vi "Project 5 Help 2.vi"() -> ()   [LabVIEW 2019]
panel:
  in  "stop":bool
  in  "stop (F)":bool
  out "size(s)":i32
  in  "Sim Mode":bool
  in  "Read File":bool
  out "Array":dbl[](array[numeric])
  out "Time":dynamicdata(graph)
  out "Data":dynamicdata(graph)
  out "Waveform Graph":waveform(dbl)(graph)
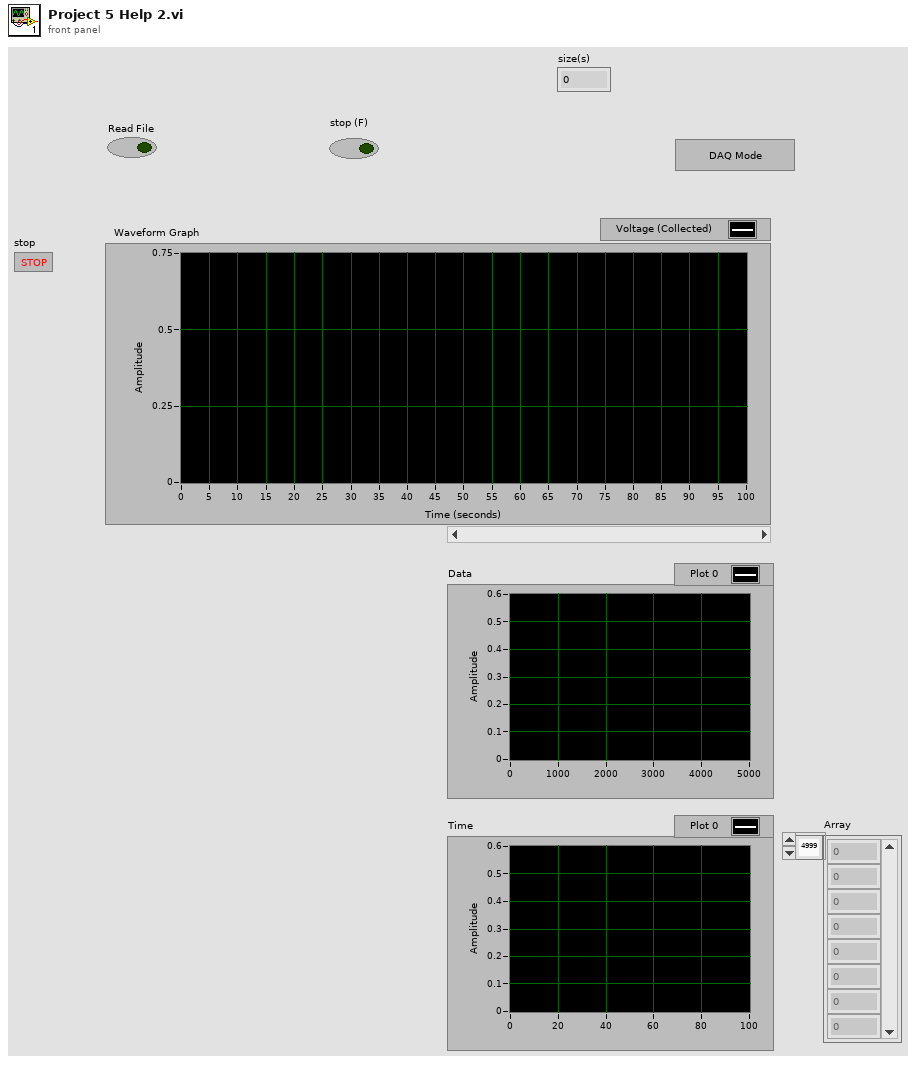
[diagram p1: front panel]
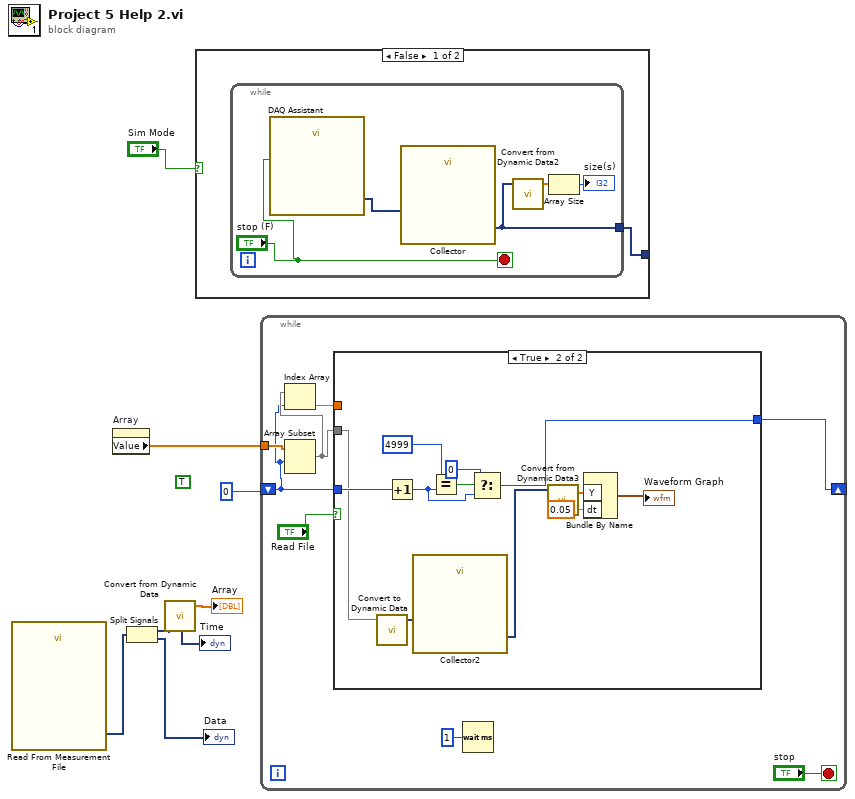
[diagram p0: block diagram]
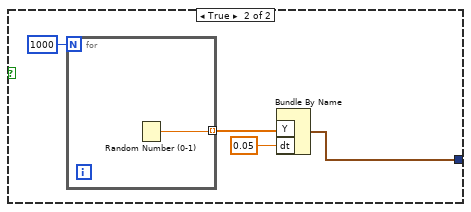
[diagram p3: hidden frame]
diagram:
  (unwired) TRUE ("EOF?")
  n1 = call "Read From Measurement File"() -> ("Signals"=w3:dynamicdata)  [unwired: 6 in, 5 out]
  n2 = property on="Array" class="Arr (strict)"() -> ("Value"=w2:dbl[])  [unwired: 2 in, 2 out]
  n3 = Split Signals(w3) -> (w5:dynamicdata, →"Data":dynamicdata)  [unwired: 2 in]
  "Time" <- w5
  n4 = call "Convert from Dynamic Data"("Dynamic Data Type"=w5) -> ("Array"=→"Array":dbl[])  [unwired: 3 in]
  n5 = case shown="False" "Sim Mode" {
    tunnel: [w8 w14] -> _
    frame False {
      n6 = while {
        tunnel: [w13] -> w8
        stop <- "stop (F)" stop-if-true
        n7 = call "DAQ Assistant"("stop (F)"="stop (F)") -> ("data"=w10:dynamicdata)  [unwired: 15 in, 3 out]
        n8 = call "Collector"("Signals"=w10) -> ("Collected Signals"=w13:dynamicdata)  [unwired: 9 in, 1 out]
        n9 = call "Convert from Dynamic Data2"("Dynamic Data Type"=w13) -> ("Array"=w11:dbl[])  [unwired: 3 in]
        n10 = Array Size(array=w11) -> (size(s)=→"size(s)":i32)
      }
    }
    frame True {
      n11 = for {
        N: 1000 -> [_]
        tunnel: [w18] -> w15 mode=indexing
        n12 = Random Number (0-1)() -> (number: 0 to 1=w18:dbl)
      }
      n13 = Bundle By Name("Y"=w15, "dt"=0.05) -> (w14:waveform(dbl))  [unwired: 1 in]
    }
  }
  n14 = while {
    tunnel: w2 -> [w24]
    shift-right: [w23] -> _
    shift-left: 0 -> [w20]
    stop <- "stop" stop-if-true
    n15 = Array Subset(array=w24, index=w20) -> (w22:dbl[])  [unwired: 1 in]
    n16 = Index Array(array=w22, index=w20) -> (element=w19:dbl)
    n17 = case shown="True" "Read File" {
      tunnel: [w27 w34] -> w23
      tunnel: w20 -> [w27 w38]
      tunnel: w22 -> [_ w28]
      tunnel: w19 -> [_ _]
      frame False {
      }
      frame True {
        n18 = call "Convert to Dynamic Data"("Array"=w28) -> ("Dynamic Data Type"=w31:dynamicdata)  [unwired: 3 in]
        n19 = Increment(x=w38) -> (x+1=w35:i32)
        n20 = call "Collector2"("Signals"=w31) -> ("Collected Signals"=w30:dynamicdata)  [unwired: 9 in, 1 out]
        n21 = Equal?(x=4999, y=w35) -> (x = y?=w36:bool)
        n22 = Select(t=0, s=w36, f=w35) -> (s? t:f=w34:i32)
        n23 = call "Convert from Dynamic Data3"("Dynamic Data Type"=w30) -> ("Array"=w29:dbl[])  [unwired: 3 in]
        n24 = Bundle By Name("Y"=w29, "dt"=0.05) -> (→"Waveform Graph":waveform(dbl))  [unwired: 1 in]
      }
    }
    n25 = Wait (ms)(milliseconds to wait=u32 1) -> ()  [unwired: 1 out]
  }
